vi "Do Request.vi"(7 "Processing In":refnum<class "Processing.lvclass">, 11 "Test Index in":refnum<class "Test Index.lvclass">) -> (0 "error out":errorcluster, 5 "Processing":refnum<class "Processing.lvclass">)   [LabVIEW 2020, in "Test Index.lvclass"]
uses:
  Test Index.lvclass
  <vilib>/IlluminatedG/IG HTTP Server/HTTP Server/Processing/Processing.lvclass
  <vilib>/IlluminatedG/IG HTTP Server/HTTP Server/Processing/Processing.lvclass/Processing.ctl
  <vilib>/IlluminatedG/IG HTTP Server/HTTP Server/Values/Values.lvclass
  <vilib>/IlluminatedG/IG HTTP Utils/HTTP Utils/Response/Response.lvclass
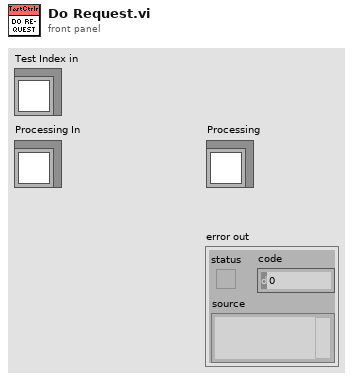
[diagram p1: front panel]
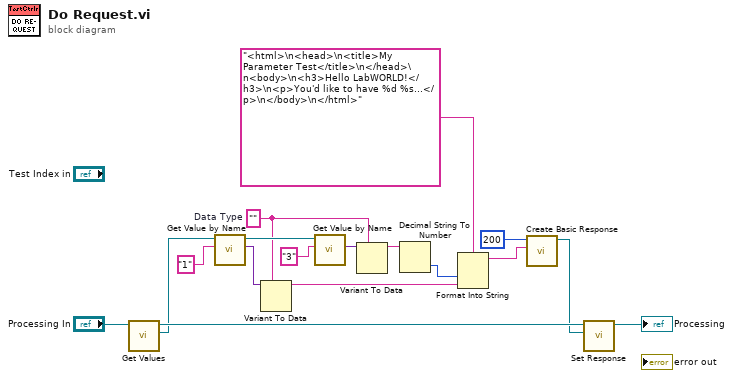
[diagram p0: block diagram]
diagram:
  w2 = ""  # Data Type
  n1 = call <vilib>:"Get Values.vi"("Processing in"="Processing In") -> ("Values"=w9:refnum<class "Values.lvclass">, "Processing out"=w12:refnum<class "Processing.lvclass">)  [unwired: 9 in]
  n2 = call <vilib>:"Get Value by Name.vi"("Name"="1" ("Name for Type (Service)"), "Values in"=w9) -> ("Value"=w6:variant, "Values out"=w4:refnum<class "Values.lvclass">)  [unwired: 7 in, 1 out]
  n3 = Variant To Data(type=w2, Variant=w6) -> (data=w7:string)  [unwired: 1 in, 1 out]
  n4 = call <vilib>:"Get Value by Name.vi"("Name"="3" ("Name for Type (Service)"), "Values in"=w4) -> ("Value"=w3:variant)  [unwired: 7 in, 2 out]
  n5 = Variant To Data(type=w2, Variant=w3) -> (data=w1:string)  [unwired: 1 in, 1 out]
  n6 = Decimal String To Number(string=w1) -> (number=w16:i32)  [unwired: 2 in, 1 out]
  n7 = Format Into String(format string="<html>\n<head>\n<title>My Parameter Test</title>\n</head>\n<body>\n<h3>Hello LabWORLD!</h3>\n<p>You'd like to have %d %s...</p>\n</body>\n</html>", w16, w7) -> (resulting string=w15:string)  [unwired: 2 in, 1 out]
  n8 = call <vilib>:"Create Basic Response.vi"("Payload"=w15, "Status Code"=u16 200) -> ("Response out"=w10:refnum<class "Response.lvclass">)  [unwired: 8 in, 1 out]
  n9 = call <vilib>:"Set Response.vi"("Response"=w10, "Processing in"=w12) -> ("Processing out"=→"Processing":refnum<class "Processing.lvclass">)  [unwired: 9 in]
